vi "通讯.vi"() -> ()   [LabVIEW 2016, in "LDM51明渠流量计.lvlib"]
uses:
  <vilib>/Analysis/baseanly.llb/Mean (DBL).vi
  <vilib>/Plasmionique/MB Master/MB_Master_Serial/MB_Master_Serial.lvclass
  C:/Program Files (x86)/National Instruments/LabVIEW 2016/vi.lib/Plasmionique/MB Master/MB_Master/MB_Master.lvclass
  <vilib>/Plasmionique/MB Master/MB Master.lvlib
  <vilib>/Analysis/NI_AALBase.lvlib
panel:
  out "总累积流量":dbl
  out "总流量":dbl
  out "平均流速":dbl
  out "平均水位":dbl
  out "累积流量":u32[](array[numeric])
  out "流速":dbl[](array[numeric])
  out "流量":dbl[](array[numeric])
  out "水位":dbl[](array[numeric])
  out "流量计启用":bool[](array[boolean])
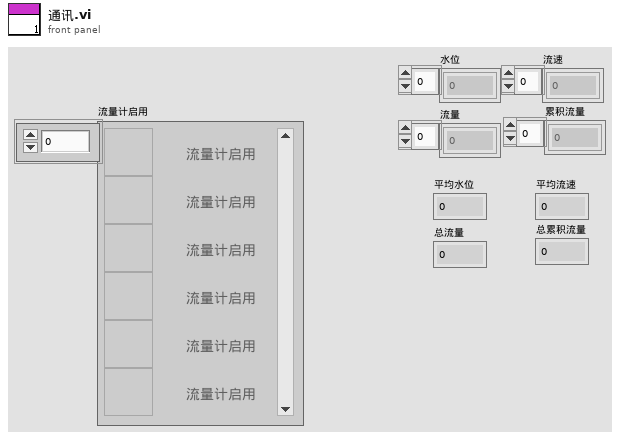
[diagram p1: front panel]
types:
  T1 = cluster{"baud rate (bps)":u32, "stop bits":u16, "parity":u16, "flow control":u16, "timeout":u32, "retries":i32}
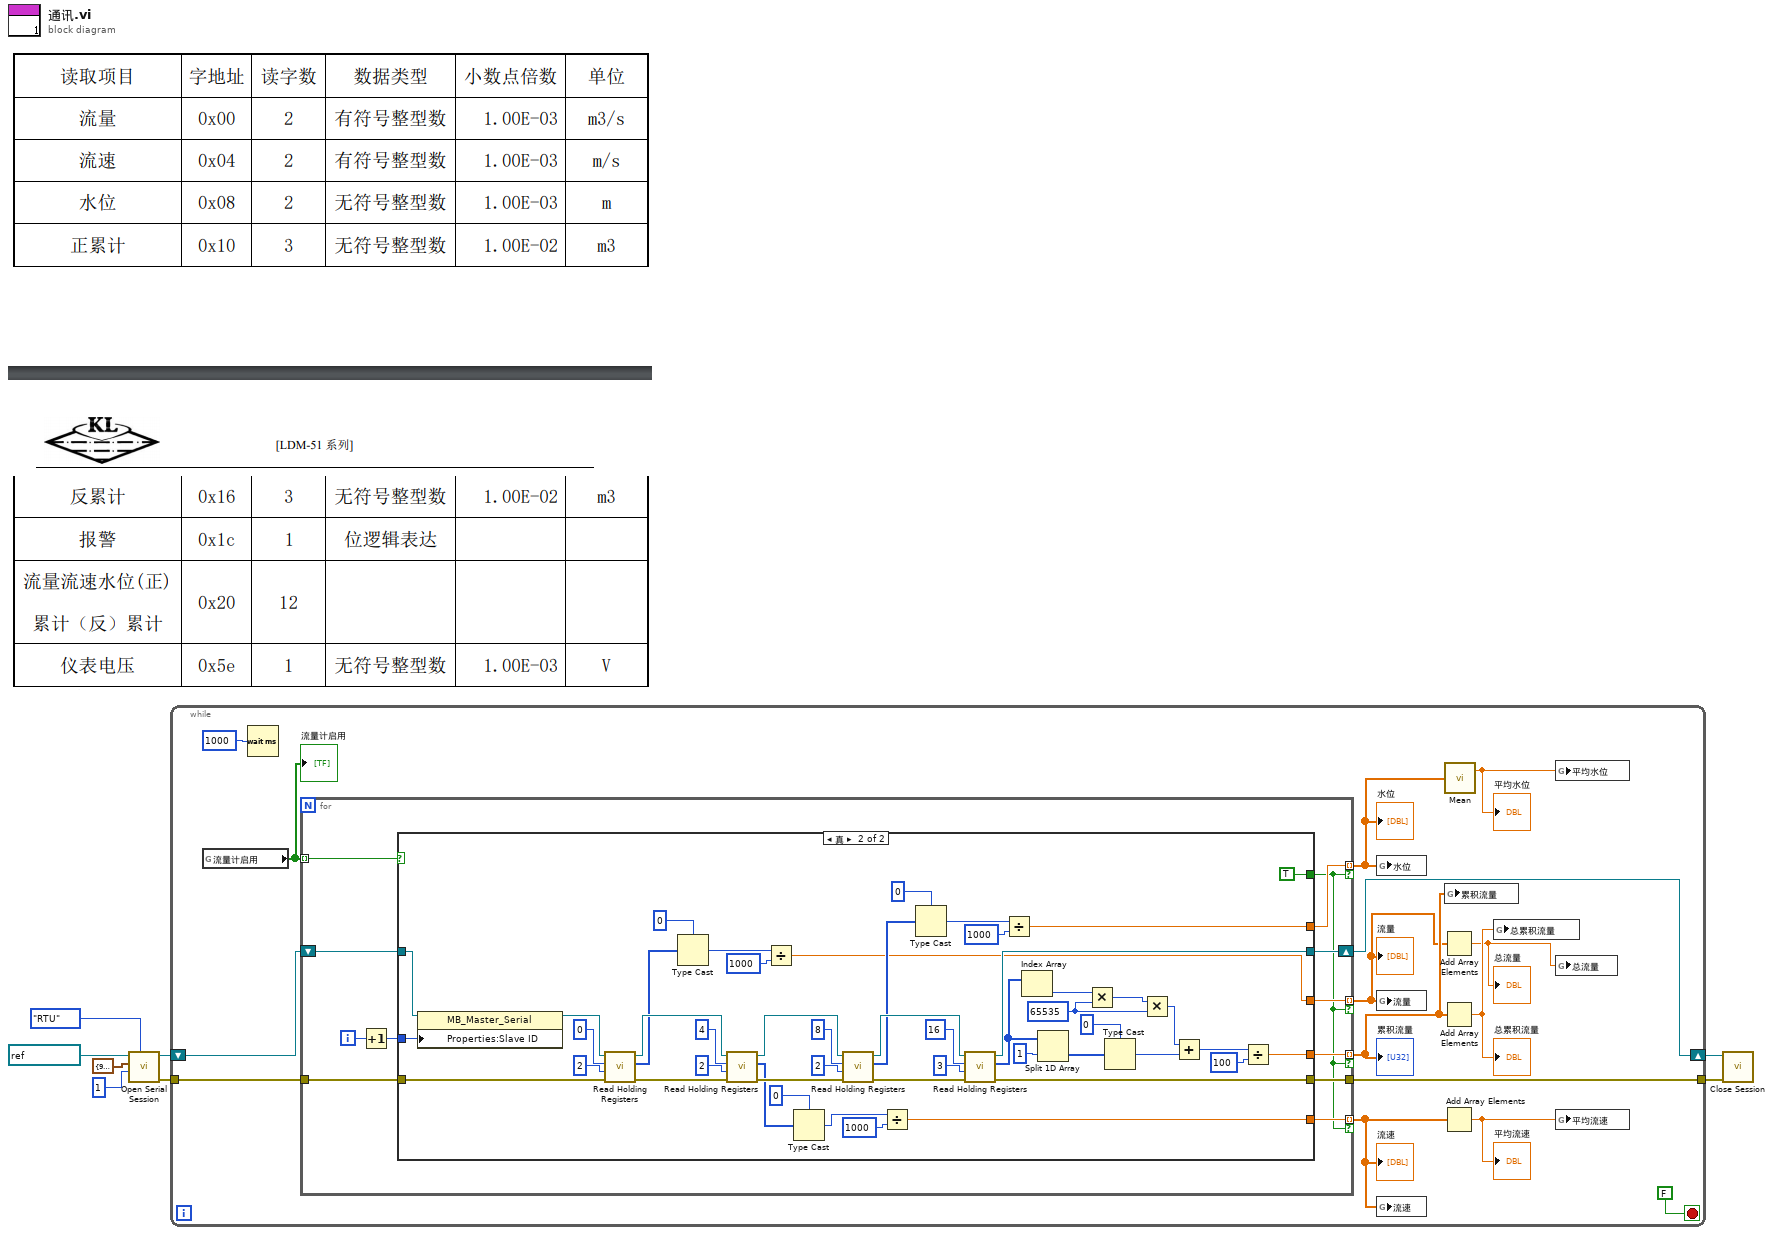
[diagram p0: block diagram]
diagram:
  n1 = call <vilib>:"Open Serial Session.vi"("Mode (RTU)"=enum16{"RTU", "ASCII"}."RTU", "Slave ID"=u8 1, "Serial Config"=T1 {"baud rate (bps)"=9600, "stop bits"=10, "parity"=0, "flow control"=0, "timeout"=1000, "retries"=1}, "VISA Resource"=refnum<visa-resource-name> "COM10") -> ("Error out"=w6:errorcluster, "MB_Serial session"=w1:refnum<class "MB_Master_Serial.lvclass">)  [unwired: 6 in]
  n2 = while {
    tunnel: w6 -> [w23]
    shift-right: [w22] -> w8
    shift-left: w1 -> [w18]
    tunnel: [w21] -> w7
    stop <- FALSE stop-if-true
    n3 = global read "LDM51全局变量.vi" "流量计启用"() -> (w11:bool[])
    "流量计启用" <- w11
    n4 = Wait (ms)(milliseconds to wait=u32 1000 ("等待时间（毫秒）")) -> ()  [unwired: 1 out]
    n5 = for {
      shift-right: [w34] -> w22
      shift-left: w18 -> [w32]
      tunnel: w11 -> [w29] mode=indexing
      tunnel: [w28] -> w15 mode=indexing if=w24
      tunnel: [w27] -> w17 mode=indexing if=w24
      tunnel: [w26] -> w16 mode=indexing if=w24
      tunnel: [w25] -> w10 mode=indexing if=w24
      tunnel: w23 -> [w35]
      tunnel: [w33] -> w21
      i -> [w31]
      n6 = Increment(x=w31) -> (x+1=w30:i32)
      n7 = case shown="真" w29 {
        tunnel: w35 -> [w36 w85]
        tunnel: [w37 w71] -> w34
        tunnel: [w36 w70] -> w33
        tunnel: w32 -> [w37 w59]
        tunnel: w30 -> [_ w57]
        tunnel: [_ w56] -> w28
        tunnel: [_ w55] -> w27
        tunnel: [_ w38] -> w26
        tunnel: [_ w54] -> w25
        tunnel: [_ TRUE] -> w24
        frame False {
        }
        frame True {
          w42 = u32 65535 ("y")
          n8 = property class="MB_Master_Serial"(reference=w59, "Properties:Slave ID"=w57) -> (reference out=w58:refnum<class "MB_Master_Serial.lvclass">)  [unwired: 1 in, 1 out]
          n9 = call <vilib>:"Read Holding Registers.vi"("error in (no error)"=w85, "quantity"=u16 2, "starting address"=u16 0, "MB session in"=w58) -> ("error out"=w81:errorcluster, "Registers"=w69:u16[], "MB session out"=w82:refnum<class "MB_Master_Serial.lvclass">)  [unwired: 5 in]
          n10 = Type Cast(type=0, x=w69) -> (*(type *) &x=w53:i32)
          n11 = call <vilib>:"Read Holding Registers.vi"("error in (no error)"=w81, "quantity"=u16 2, "starting address"=u16 4, "MB session in"=w82) -> ("error out"=w75:errorcluster, "Registers"=w68:u16[], "MB session out"=w78:refnum<class "MB_Master_Serial.lvclass">)  [unwired: 5 in]
          n12 = Divide(x=w53, y=1000) -> (x/y=w56:dbl)
          n13 = Type Cast(type=0, x=w68) -> (*(type *) &x=w51:i32)
          n14 = call <vilib>:"Read Holding Registers.vi"("error in (no error)"=w75, "quantity"=u16 2, "starting address"=u16 8, "MB session in"=w78) -> ("error out"=w73:errorcluster, "Registers"=w66:u16[], "MB session out"=w74:refnum<class "MB_Master_Serial.lvclass">)  [unwired: 5 in]
          n15 = Divide(x=w51, y=1000) -> (x/y=w54:dbl)
          n16 = Type Cast(type=0, x=w66) -> (*(type *) &x=w52:i32)
          n17 = call <vilib>:"Read Holding Registers.vi"("error in (no error)"=w73, "quantity"=u16 3, "starting address"=u16 16, "MB session in"=w74) -> ("error out"=w70:errorcluster, "Registers"=w49:u16[], "MB session out"=w71:refnum<class "MB_Master_Serial.lvclass">)  [unwired: 5 in]
          n18 = Divide(x=w52, y=1000) -> (x/y=w55:dbl)
          n19 = Index Array(array=w49) -> (element=w44:u16)  [unwired: 1 in]
          n20 = Split 1D Array(array=w49, index=1 ("索引")) -> (second subarray=w47:u16[])  [unwired: 1 out]
          n21 = Multiply(x=w44, y=w42) -> (x*y=w43:u32)
          n22 = Type Cast(type=0, x=w47) -> (*(type *) &x=w45:i32)
          n23 = Multiply(x=w43, y=w42) -> (x*y=w41:u32)
          n24 = Add(x=w41, y=w45) -> (x+y=w40:u32)
          n25 = Divide(x=w40, y=100) -> (x/y=w38:dbl)
        }
      }
    }
    "水位" <- w17
    "流量" <- w15
    "流速" <- w10
    "累积流量" <- w16
    n26 = global write "LDM51全局变量.vi" "水位"(w17) -> ()
    n27 = global write "LDM51全局变量.vi" "流量"(w15) -> ()
    n28 = global write "LDM51全局变量.vi" "流速"(w10) -> ()
    n29 = Add Array Elements(numeric array=w15) -> (sum=w12:dbl)
    "总流量" <- w12
    n30 = Add Array Elements(numeric array=w16) -> (sum=w13:dbl)
    "总累积流量" <- w13
    n31 = Add Array Elements(numeric array=w10) -> (sum=w9:dbl)
    "平均流速" <- w9
    n32 = call-poly <vilib>:"Mean.vi"("X"=w17) -> ("mean"=w14:dbl)  [unwired: 1 out]
    "平均水位" <- w14
    n33 = global write "LDM51全局变量.vi" "累积流量"(w16) -> ()
    n34 = global write "LDM51全局变量.vi" "总累积流量"(w13) -> ()
    n35 = global write "LDM51全局变量.vi" "平均水位"(w14) -> ()
    n36 = global write "LDM51全局变量.vi" "总流量"(w12) -> ()
    n37 = global write "LDM51全局变量.vi" "平均流速"(w9) -> ()
  }
  n38 = call-dynamic "Close Session.vi"("error in (no error)"=w7, "MB_Serial session"=w8) -> ()  [unwired: 9 in, 1 out]
